vi "Write value to memory.vi"(8 "error in (no error)":errorcluster, 9 "Index":i32, 10 "Value":string, 11 "Data Type":T1) -> (0 "error out":errorcluster)   [LabVIEW 2020, in "Current Value Table(Rebuild).lvlib"]
uses:
  Current Value Table(Rebuild).lvlib
  Type Defs/Data Types.ctl
  Type Defs/Memory Commands.ctl
  DataTypes/Double_ASCII String To Data.vi
  DataTypes/Array of String_ASCII String To Data.vi
  DataTypes/Array of Boolean_ASCII String To Data.vi
  DataTypes/Array of Single_ASCII String To Data.vi
  DataTypes/Array of Double_ASCII String To Data.vi
  DataTypes/Array of I8_ASCII String To Data.vi
  DataTypes/Array of I16_ASCII String To Data.vi
  DataTypes/Array of I32_ASCII String To Data.vi
  DataTypes/Array of I64_ASCII String To Data.vi
  DataTypes/Array of U64_ASCII String To Data.vi
  DataTypes/Array of U32_ASCII String To Data.vi
  DataTypes/Array of U16_ASCII String To Data.vi
  DataTypes/Array of U8_ASCII String To Data.vi
  DataTypes/Boolean_ASCII String To Data.vi
  DataTypes/String_ASCII String To Data.vi
  DataTypes/U8_ASCII String To Data.vi
  DataTypes/U16_ASCII String To Data.vi
  DataTypes/U32_ASCII String To Data.vi
  DataTypes/U64_ASCII String To Data.vi
  DataTypes/I8_ASCII String To Data.vi
  DataTypes/I16_ASCII String To Data.vi
  DataTypes/I32_ASCII String To Data.vi
  DataTypes/I64_ASCII String To Data.vi
  DataTypes/Single_ASCII String To Data.vi
  Errors/Scanned Value Error.vi
  Errors/Generate Error.vi
  DataTypes/Double_Memory Block.vi
  DataTypes/Array of String_Memory Block.vi
  DataTypes/Array of Boolean_Memory Block.vi
  DataTypes/Array of Single_Memory Block.vi
  DataTypes/Array of Double_Memory Block.vi
  DataTypes/Array of I8_Memory Block.vi
  DataTypes/Array of I16_Memory Block.vi
  DataTypes/Array of I32_Memory Block.vi
  DataTypes/Array of I64_Memory Block.vi
  DataTypes/Array of U64_Memory Block.vi
  DataTypes/Array of U32_Memory Block.vi
  DataTypes/Array of U16_Memory Block.vi
  DataTypes/Array of U8_Memory Block.vi
  DataTypes/Boolean_Memory Block.vi
  DataTypes/String_Memory Block.vi
  DataTypes/U8_Memory Block.vi
  DataTypes/U16_Memory Block.vi
  DataTypes/U32_Memory Block.vi
  DataTypes/U64_Memory Block.vi
  DataTypes/I8_Memory Block.vi
  DataTypes/I16_Memory Block.vi
  DataTypes/I32_Memory Block.vi
  DataTypes/I64_Memory Block.vi
  DataTypes/Single_Memory Block.vi
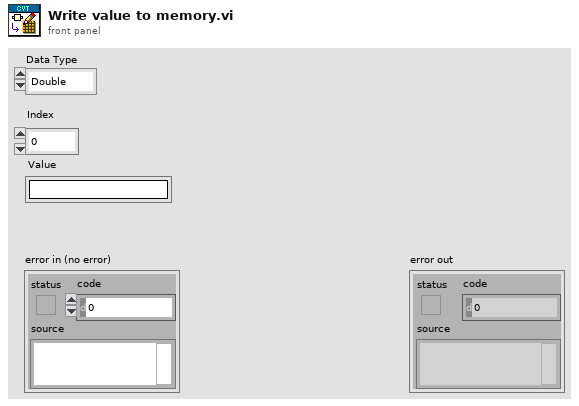
[diagram p1: front panel]
types:
  T1 = typedef "Current Value Table(Rebuild).lvlib/Data Types.ctl" = enum16{"Double", "Single", "I64", "I32", "I16", "I8", "U64", "U32", "U16", "U8", "String", "Boolean", "Array of U8", "Array of U16", "Array of U32", "Array of U64", "Array of I64", "Array of I32", "Array of I16", "Array of I8", "Array of Double", "Array of Single", "Array of Boolean", "Array of String"}
  T2 = typedef "Current Value Table(Rebuild).lvlib/Memory Commands.ctl" = enum16{"Init", "Add Data", "Read", "Read Group", "Read All", "Write", "Write Group", "Get Size"}
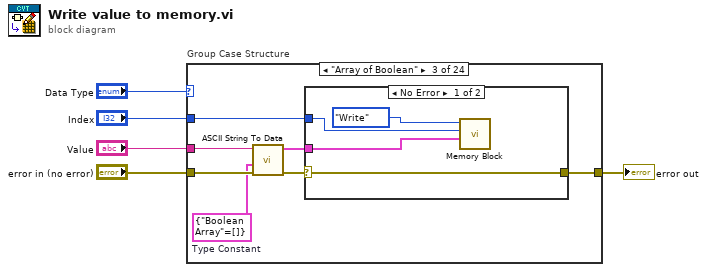
[diagram p0: block diagram]
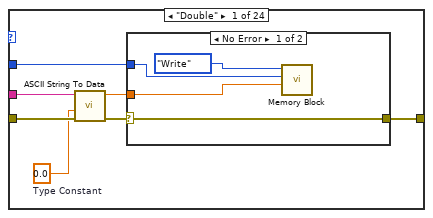
[diagram p2: hidden frame]
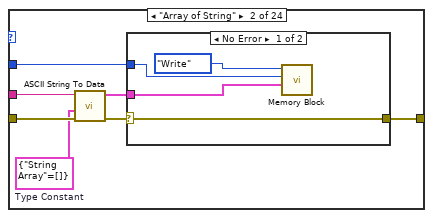
[diagram p4: hidden frame]
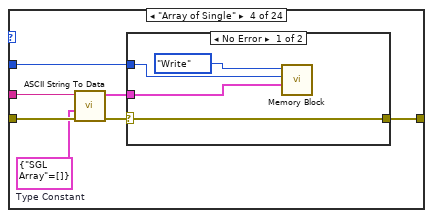
[diagram p7: hidden frame]
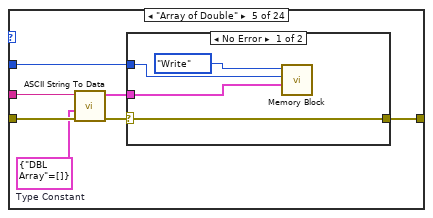
[diagram p9: hidden frame]
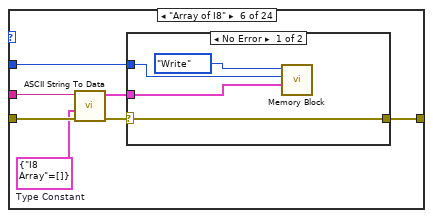
[diagram p11: hidden frame]
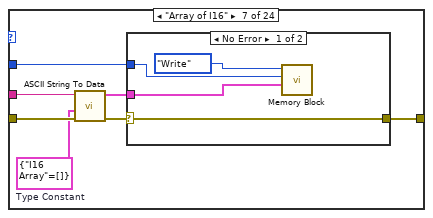
[diagram p13: hidden frame]
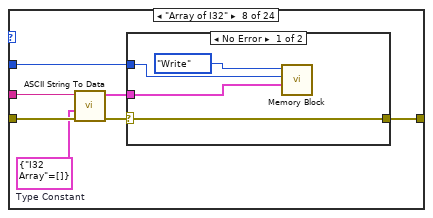
[diagram p15: hidden frame]
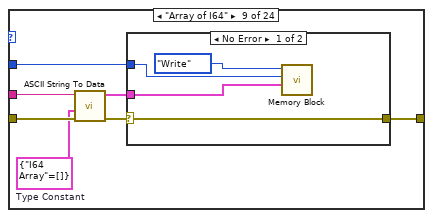
[diagram p17: hidden frame]
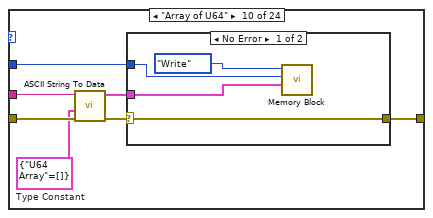
[diagram p19: hidden frame]
diagram:
  n1 = case "Group Case Structure" shown="\"Array of Boolean\"" "Data Type" {
    tunnel: "error in (no error)" -> [w12 w24 w36 w48 w60 w72 w84 w96 w108 w120 w132 w144 w156 w168 w180 w192 w204 w216 w228 w240 w252 w264 w276 w288]
    tunnel: "Value" -> [w11 w23 w35 w47 w59 w71 w83 w95 w107 w119 w131 w143 w155 w167 w179 w191 w203 w215 w227 w239 w251 w263 w275 w287]
    tunnel: [w9 w21 w33 w45 w57 w69 w81 w93 w105 w117 w129 w141 w153 w165 w177 w189 w201 w213 w225 w237 w249 w261 w273 w285] -> w2
    tunnel: "Index" -> [w7 w19 w31 w43 w55 w67 w79 w91 w103 w115 w127 w139 w151 w163 w175 w187 w199 w211 w223 w235 w247 w259 w271 w283]
    frame "Double" {
      w6 = 0.0  # Type Constant
      n2 = call-poly "ASCII String To Data.vi"("error in (no error)"=w12, "Default"=w6, "Value"=w11) -> ("error out"=w10:errorcluster, "Data"=w8:dbl)  [unwired: 7 in]
      n3 = case shown="No Error" w10 {
        selector: w10 -> [w15 w17]
        tunnel: w8 -> [w14 _]
        tunnel: [w15 w17] -> w9
        tunnel: w7 -> [w13 _]
        frame No Error {
          n4 = call-poly "Memory Block.vi"("Value"=w14, "Index"=w13, "Method"=Memory_Commands."Write") -> ()  [unwired: 6 in, 3 out]
        }
        frame Error {
        }
      }
    }
    frame "Array of String" {
      w18 = cluster{"String Array":string[]} {"String Array"=[]}  # Type Constant
      n5 = call-poly "ASCII String To Data.vi"("error in (no error)"=w24, "Default"=w18, "Value"=w23) -> ("error out"=w22:errorcluster, "Data"=w20:cluster{"String Array":string[]})  [unwired: 7 in]
      n6 = case shown="No Error" w22 {
        selector: w22 -> [w27 w29]
        tunnel: w20 -> [w26 _]
        tunnel: [w27 w29] -> w21
        tunnel: w19 -> [w25 _]
        frame No Error {
          n7 = call-poly "Memory Block.vi"("Value"=w26, "Index"=w25, "Method"=Memory_Commands."Write") -> ()  [unwired: 6 in, 3 out]
        }
        frame Error {
        }
      }
    }
    frame "Array of Boolean" {
      w30 = cluster{"Boolean Array":bool[]} {"Boolean Array"=[]}  # Type Constant
      n8 = call-poly "ASCII String To Data.vi"("error in (no error)"=w36, "Default"=w30, "Value"=w35) -> ("error out"=w34:errorcluster, "Data"=w32:cluster{"Boolean Array":bool[]})  [unwired: 7 in]
      n9 = case shown="No Error" w34 {
        selector: w34 -> [w39 w41]
        tunnel: w32 -> [w38 _]
        tunnel: [w39 w41] -> w33
        tunnel: w31 -> [w37 _]
        frame No Error {
          n10 = call-poly "Memory Block.vi"("Value"=w38, "Index"=w37, "Method"=Memory_Commands."Write") -> ()  [unwired: 6 in, 3 out]
        }
        frame Error {
        }
      }
    }
    frame "Array of Single" {
      w42 = cluster{"SGL Array":sgl[]} {"SGL Array"=[]}  # Type Constant
      n11 = call-poly "ASCII String To Data.vi"("error in (no error)"=w48, "Default"=w42, "Value"=w47) -> ("error out"=w46:errorcluster, "Data"=w44:cluster{"SGL Array":sgl[]})  [unwired: 7 in]
      n12 = case shown="No Error" w46 {
        selector: w46 -> [w51 w53]
        tunnel: w44 -> [w50 _]
        tunnel: [w51 w53] -> w45
        tunnel: w43 -> [w49 _]
        frame No Error {
          n13 = call-poly "Memory Block.vi"("Value"=w50, "Index"=w49, "Method"=Memory_Commands."Write") -> ()  [unwired: 6 in, 3 out]
        }
        frame Error {
        }
      }
    }
    frame "Array of Double" {
      w54 = cluster{"DBL Array":dbl[]} {"DBL Array"=[]}  # Type Constant
      n14 = call-poly "ASCII String To Data.vi"("error in (no error)"=w60, "Default"=w54, "Value"=w59) -> ("error out"=w58:errorcluster, "Data"=w56:cluster{"DBL Array":dbl[]})  [unwired: 7 in]
      n15 = case shown="No Error" w58 {
        selector: w58 -> [w63 w65]
        tunnel: w56 -> [w62 _]
        tunnel: [w63 w65] -> w57
        tunnel: w55 -> [w61 _]
        frame No Error {
          n16 = call-poly "Memory Block.vi"("Value"=w62, "Index"=w61, "Method"=Memory_Commands."Write") -> ()  [unwired: 6 in, 3 out]
        }
        frame Error {
        }
      }
    }
    frame "Array of I8" {
      w66 = cluster{"I8 Array":i8[]} {"I8 Array"=[]}  # Type Constant
      n17 = call-poly "ASCII String To Data.vi"("error in (no error)"=w72, "Default"=w66, "Value"=w71) -> ("error out"=w70:errorcluster, "Data"=w68:cluster{"I8 Array":i8[]})  [unwired: 7 in]
      n18 = case shown="No Error" w70 {
        selector: w70 -> [w75 w77]
        tunnel: w68 -> [w74 _]
        tunnel: [w75 w77] -> w69
        tunnel: w67 -> [w73 _]
        frame No Error {
          n19 = call-poly "Memory Block.vi"("Value"=w74, "Index"=w73, "Method"=Memory_Commands."Write") -> ()  [unwired: 6 in, 3 out]
        }
        frame Error {
        }
      }
    }
    frame "Array of I16" {
      w78 = cluster{"I16 Array":i16[]} {"I16 Array"=[]}  # Type Constant
      n20 = call-poly "ASCII String To Data.vi"("error in (no error)"=w84, "Default"=w78, "Value"=w83) -> ("error out"=w82:errorcluster, "Data"=w80:cluster{"I16 Array":i16[]})  [unwired: 7 in]
      n21 = case shown="No Error" w82 {
        selector: w82 -> [w87 w89]
        tunnel: w80 -> [w86 _]
        tunnel: [w87 w89] -> w81
        tunnel: w79 -> [w85 _]
        frame No Error {
          n22 = call-poly "Memory Block.vi"("Value"=w86, "Index"=w85, "Method"=Memory_Commands."Write") -> ()  [unwired: 6 in, 3 out]
        }
        frame Error {
        }
      }
    }
    frame "Array of I32" {
      w90 = cluster{"I32 Array":i32[]} {"I32 Array"=[]}  # Type Constant
      n23 = call-poly "ASCII String To Data.vi"("error in (no error)"=w96, "Default"=w90, "Value"=w95) -> ("error out"=w94:errorcluster, "Data"=w92:cluster{"I32 Array":i32[]})  [unwired: 7 in]
      n24 = case shown="No Error" w94 {
        selector: w94 -> [w99 w101]
        tunnel: w92 -> [w98 _]
        tunnel: [w99 w101] -> w93
        tunnel: w91 -> [w97 _]
        frame No Error {
          n25 = call-poly "Memory Block.vi"("Value"=w98, "Index"=w97, "Method"=Memory_Commands."Write") -> ()  [unwired: 6 in, 3 out]
        }
        frame Error {
        }
      }
    }
    frame "Array of I64" {
      w102 = cluster{"I64 Array":i64[]} {"I64 Array"=[]}  # Type Constant
      n26 = call-poly "ASCII String To Data.vi"("error in (no error)"=w108, "Default"=w102, "Value"=w107) -> ("error out"=w106:errorcluster, "Data"=w104:cluster{"I64 Array":i64[]})  [unwired: 7 in]
      n27 = case shown="No Error" w106 {
        selector: w106 -> [w111 w113]
        tunnel: w104 -> [w110 _]
        tunnel: [w111 w113] -> w105
        tunnel: w103 -> [w109 _]
        frame No Error {
          n28 = call-poly "Memory Block.vi"("Value"=w110, "Index"=w109, "Method"=Memory_Commands."Write") -> ()  [unwired: 6 in, 3 out]
        }
        frame Error {
        }
      }
    }
    frame "Array of U64" {
      w114 = cluster{"U64 Array":u64[]} {"U64 Array"=[]}  # Type Constant
      n29 = call-poly "ASCII String To Data.vi"("error in (no error)"=w120, "Default"=w114, "Value"=w119) -> ("error out"=w118:errorcluster, "Data"=w116:cluster{"U64 Array":u64[]})  [unwired: 7 in]
      n30 = case shown="No Error" w118 {
        selector: w118 -> [w123 w125]
        tunnel: w116 -> [w122 _]
        tunnel: [w123 w125] -> w117
        tunnel: w115 -> [w121 _]
        frame No Error {
          n31 = call-poly "Memory Block.vi"("Value"=w122, "Index"=w121, "Method"=Memory_Commands."Write") -> ()  [unwired: 6 in, 3 out]
        }
        frame Error {
        }
      }
    }
    frame "Array of U32" {
      w126 = cluster{"U32 Array":u32[]} {"U32 Array"=[]}  # Type Constant
      n32 = call-poly "ASCII String To Data.vi"("error in (no error)"=w132, "Default"=w126, "Value"=w131) -> ("error out"=w130:errorcluster, "Data"=w128:cluster{"U32 Array":u32[]})  [unwired: 7 in]
      n33 = case shown="No Error" w130 {
        selector: w130 -> [w135 w137]
        tunnel: w128 -> [w134 _]
        tunnel: [w135 w137] -> w129
        tunnel: w127 -> [w133 _]
        frame No Error {
          n34 = call-poly "Memory Block.vi"("Value"=w134, "Index"=w133, "Method"=Memory_Commands."Write") -> ()  [unwired: 6 in, 3 out]
        }
        frame Error {
        }
      }
    }
    frame "Array of U16" {
      w138 = cluster{"U16 Array":u16[]} {"U16 Array"=[]}  # Type Constant
      n35 = call-poly "ASCII String To Data.vi"("error in (no error)"=w144, "Default"=w138, "Value"=w143) -> ("error out"=w142:errorcluster, "Data"=w140:cluster{"U16 Array":u16[]})  [unwired: 7 in]
      n36 = case shown="No Error" w142 {
        selector: w142 -> [w147 w149]
        tunnel: w140 -> [w146 _]
        tunnel: [w147 w149] -> w141
        tunnel: w139 -> [w145 _]
        frame No Error {
          n37 = call-poly "Memory Block.vi"("Value"=w146, "Index"=w145, "Method"=Memory_Commands."Write") -> ()  [unwired: 6 in, 3 out]
        }
        frame Error {
        }
      }
    }
    frame "Array of U8" {
      w150 = cluster{"U8 Array":u8[]} {"U8 Array"=[]}  # Type Constant
      n38 = call-poly "ASCII String To Data.vi"("error in (no error)"=w156, "Default"=w150, "Value"=w155) -> ("error out"=w154:errorcluster, "Data"=w152:cluster{"U8 Array":u8[]})  [unwired: 7 in]
      n39 = case shown="No Error" w154 {
        selector: w154 -> [w159 w161]
        tunnel: w152 -> [w158 _]
        tunnel: [w159 w161] -> w153
        tunnel: w151 -> [w157 _]
        frame No Error {
          n40 = call-poly "Memory Block.vi"("Value"=w158, "Index"=w157, "Method"=Memory_Commands."Write") -> ()  [unwired: 6 in, 3 out]
        }
        frame Error {
        }
      }
    }
    frame "Boolean" {
      w162 = FALSE  # bool
      n41 = call-poly "ASCII String To Data.vi"("error in (no error)"=w168, "Default"=w162, "Value"=w167) -> ("error out"=w166:errorcluster, "Data"=w164:bool)  [unwired: 7 in]
      n42 = case shown="No Error" w166 {
        selector: w166 -> [w171 w173]
        tunnel: w164 -> [w170 _]
        tunnel: [w171 w173] -> w165
        tunnel: w163 -> [w169 _]
        frame No Error {
          n43 = call-poly "Memory Block.vi"("Value"=w170, "Index"=w169, "Method"=Memory_Commands."Write") -> ()  [unwired: 6 in, 3 out]
        }
        frame Error {
        }
      }
    }
    frame "String" {
      w174 = ""  # Type Constant
      n44 = call-poly "ASCII String To Data.vi"("error in (no error)"=w180, "Default"=w174, "Value"=w179) -> ("error out"=w178:errorcluster, "Data"=w176:string)  [unwired: 7 in]
      n45 = case shown="No Error" w178 {
        selector: w178 -> [w183 w185]
        tunnel: w176 -> [w182 _]
        tunnel: [w183 w185] -> w177
        tunnel: w175 -> [w181 _]
        frame No Error {
          n46 = call-poly "Memory Block.vi"("Value"=w182, "Index"=w181, "Method"=Memory_Commands."Write") -> ()  [unwired: 6 in, 3 out]
        }
        frame Error {
        }
      }
    }
    frame "U8" {
      w186 = u8 0  # Type Constant
      n47 = call-poly "ASCII String To Data.vi"("error in (no error)"=w192, "Default"=w186, "Value"=w191) -> ("error out"=w190:errorcluster, "Data"=w188:u8)  [unwired: 7 in]
      n48 = case shown="No Error" w190 {
        selector: w190 -> [w195 w197]
        tunnel: w188 -> [w194 _]
        tunnel: [w195 w197] -> w189
        tunnel: w187 -> [w193 _]
        frame No Error {
          n49 = call-poly "Memory Block.vi"("Value"=w194, "Index"=w193, "Method"=Memory_Commands."Write") -> ()  [unwired: 6 in, 3 out]
        }
        frame Error {
        }
      }
    }
    frame "U16" {
      w198 = u16 0  # Type Constant
      n50 = call-poly "ASCII String To Data.vi"("error in (no error)"=w204, "Default"=w198, "Value"=w203) -> ("error out"=w202:errorcluster, "Data"=w200:u16)  [unwired: 7 in]
      n51 = case shown="No Error" w202 {
        selector: w202 -> [w207 w209]
        tunnel: w200 -> [w206 _]
        tunnel: [w207 w209] -> w201
        tunnel: w199 -> [w205 _]
        frame No Error {
          n52 = call-poly "Memory Block.vi"("Value"=w206, "Index"=w205, "Method"=Memory_Commands."Write") -> ()  [unwired: 6 in, 3 out]
        }
        frame Error {
        }
      }
    }
    frame "U32" {
      w210 = u32 0  # Type Constant
      n53 = call-poly "ASCII String To Data.vi"("error in (no error)"=w216, "Default"=w210, "Value"=w215) -> ("error out"=w214:errorcluster, "Data"=w212:u32)  [unwired: 7 in]
      n54 = case shown="No Error" w214 {
        selector: w214 -> [w219 w221]
        tunnel: w212 -> [w218 _]
        tunnel: [w219 w221] -> w213
        tunnel: w211 -> [w217 _]
        frame No Error {
          n55 = call-poly "Memory Block.vi"("Value"=w218, "Index"=w217, "Method"=Memory_Commands."Write") -> ()  [unwired: 6 in, 3 out]
        }
        frame Error {
        }
      }
    }
    frame "U64" {
      w222 = u64 0  # Type Constant
      n56 = call-poly "ASCII String To Data.vi"("error in (no error)"=w228, "Default"=w222, "Value"=w227) -> ("error out"=w226:errorcluster, "Data"=w224:u64)  [unwired: 7 in]
      n57 = case shown="No Error" w226 {
        selector: w226 -> [w231 w233]
        tunnel: w224 -> [w230 _]
        tunnel: [w231 w233] -> w225
        tunnel: w223 -> [w229 _]
        frame No Error {
          n58 = call-poly "Memory Block.vi"("Value"=w230, "Index"=w229, "Method"=Memory_Commands."Write") -> ()  [unwired: 6 in, 3 out]
        }
        frame Error {
        }
      }
    }
    frame "I8" {
      w234 = i8 0  # Type Constant
      n59 = call-poly "ASCII String To Data.vi"("error in (no error)"=w240, "Default"=w234, "Value"=w239) -> ("error out"=w238:errorcluster, "Data"=w236:i8)  [unwired: 7 in]
      n60 = case shown="No Error" w238 {
        selector: w238 -> [w243 w245]
        tunnel: w236 -> [w242 _]
        tunnel: [w243 w245] -> w237
        tunnel: w235 -> [w241 _]
        frame No Error {
          n61 = call-poly "Memory Block.vi"("Value"=w242, "Index"=w241, "Method"=Memory_Commands."Write") -> ()  [unwired: 6 in, 3 out]
        }
        frame Error {
        }
      }
    }
    frame "I16" {
      w246 = i16 0  # Type Constant
      n62 = call-poly "ASCII String To Data.vi"("error in (no error)"=w252, "Default"=w246, "Value"=w251) -> ("error out"=w250:errorcluster, "Data"=w248:i16)  [unwired: 7 in]
      n63 = case shown="No Error" w250 {
        selector: w250 -> [w255 w257]
        tunnel: w248 -> [w254 _]
        tunnel: [w255 w257] -> w249
        tunnel: w247 -> [w253 _]
        frame No Error {
          n64 = call-poly "Memory Block.vi"("Value"=w254, "Index"=w253, "Method"=Memory_Commands."Write") -> ()  [unwired: 6 in, 3 out]
        }
        frame Error {
        }
      }
    }
    frame "I32" {
      w258 = 0  # Type Constant
      n65 = call-poly "ASCII String To Data.vi"("error in (no error)"=w264, "Default"=w258, "Value"=w263) -> ("error out"=w262:errorcluster, "Data"=w260:i32)  [unwired: 7 in]
      n66 = case shown="No Error" w262 {
        selector: w262 -> [w267 w269]
        tunnel: w260 -> [w266 _]
        tunnel: [w267 w269] -> w261
        tunnel: w259 -> [w265 _]
        frame No Error {
          n67 = call-poly "Memory Block.vi"("Value"=w266, "Index"=w265, "Method"=Memory_Commands."Write") -> ()  [unwired: 6 in, 3 out]
        }
        frame Error {
        }
      }
    }
    frame "I64" {
      w270 = i64 0  # Type Constant
      n68 = call-poly "ASCII String To Data.vi"("error in (no error)"=w276, "Default"=w270, "Value"=w275) -> ("error out"=w274:errorcluster, "Data"=w272:i64)  [unwired: 7 in]
      n69 = case shown="No Error" w274 {
        selector: w274 -> [w279 w281]
        tunnel: w272 -> [w278 _]
        tunnel: [w279 w281] -> w273
        tunnel: w271 -> [w277 _]
        frame No Error {
          n70 = call-poly "Memory Block.vi"("Value"=w278, "Index"=w277, "Method"=Memory_Commands."Write") -> ()  [unwired: 6 in, 3 out]
        }
        frame Error {
        }
      }
    }
    frame "Single" {
      w282 = sgl 0.0  # Type Constant
      n71 = call-poly "ASCII String To Data.vi"("error in (no error)"=w288, "Default"=w282, "Value"=w287) -> ("error out"=w286:errorcluster, "Data"=w284:sgl)  [unwired: 7 in]
      n72 = case shown="No Error" w286 {
        selector: w286 -> [w291 w293]
        tunnel: w284 -> [w290 _]
        tunnel: [w291 w293] -> w285
        tunnel: w283 -> [w289 _]
        frame No Error {
          n73 = call-poly "Memory Block.vi"("Value"=w290, "Index"=w289, "Method"=Memory_Commands."Write") -> ()  [unwired: 6 in, 3 out]
        }
        frame Error {
        }
      }
    }
  }
  "error out" <- w2
